vi "freq_damping_to_z.vi"(6 "Fs":dbl, 10 "Characteristics":T1 {"Frequency" format="%#_3p"; "Damping" min=0.0 max=1000.0 step=1.0 format="%#_3g"}) -> (0 "Coefficients":dbl[](array[numeric]) format="%#_3g", 2 "z location":cdb format="%#.3g", 3 "s location":cdb format="%#.3g")   [LabVIEW 2010]
uses:
  damping_freq.ctl
  <vilib>/analysis/polynomials.llb/Multiply Polynomials (CDB).vi
  <vilib>/Analysis/NI_AALPro.lvlib
panel:
  # "Damping factor"
  # "Natural frequency (Hz)"
  # "Difference equation coefficients"
  # "Sampling frequency (1/sec)"
  # "Convert complex pole or zero pair specified as damping factor and natural frequency into a discrete-time difference equation that can be used to construct filter parameters."
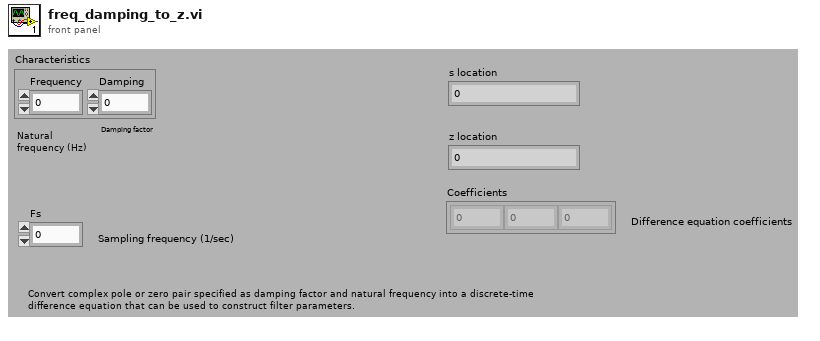
[diagram p1: front panel]
types:
  T1 = typedef "damping_freq.ctl" = cluster{"Frequency":dbl, "Damping":dbl}
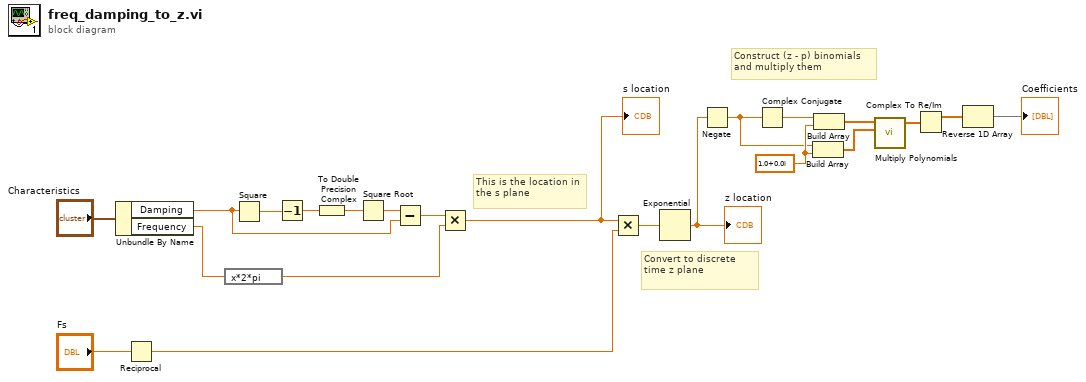
[diagram p0: block diagram]
diagram:
  w11 = cdb 1.0+0.0i ("element")
  # "Construct (z - p) binomials\nand multiply them"
  # "Convert to discrete time z plane"
  # "This is the location in the s plane"
  n1 = Unbundle By Name("Characteristics") -> ("Damping"=w4:dbl, "Frequency"=w3:dbl)
  n2 = Reciprocal(x="Fs") -> (1/x=w16:dbl)
  n3 = expression code="x*2*pi"(w3) -> (w18:dbl)
  n4 = Square(x=w4) -> (x^2=w22:dbl)
  n5 = Decrement(x=w22) -> (x-1=w21:dbl)
  n6 = To Double Precision Complex(1:w21) -> (0:w20:cdb)
  n7 = Square Root(x=w20) -> (sqrt(x)=w9:cdb)
  n8 = Subtract(x=w9, y=w4) -> (x-y=w19:cdb)
  n9 = Multiply(x=w19, y=w18) -> (x*y=w8:cdb)
  "s location" <- w8
  n10 = Multiply(x=w8, y=w16) -> (x*y=w15:cdb)
  n11 = Exponential(1:w15) -> (0:w7:cdb)
  "z location" <- w7
  n12 = Negate(x=w7) -> (-x=w6:cdb)
  n13 = Complex Conjugate(1:w6) -> (0:w14:cdb)
  n14 = Build Array(w6, w11) -> (w12:cdb[])
  n15 = Build Array(w14, w11) -> (w13:cdb[])
  n16 = call-poly <vilib>:"Multiply Polynomials.vi"("Q(x)"=w12, "P(x)"=w13) -> ("P(x)*Q(x)"=w10:cdb[])  [unwired: 2 in, 7 out]
  n17 = Complex To Re/Im(x + iy=w10) -> (x=w2:dbl[])  [unwired: 1 out]
  n18 = Reverse 1D Array(array=w2) -> (reversed array=→"Coefficients":dbl[])
